vi "Get Index.vi"(7 "item":string, 8 "error in":errorcluster, 11 "[Items]":string[](array[string])) -> (0 "error out":errorcluster, 3 "index":i32)   [LabVIEW 2024, in "LV_OPC.lvlib"]
uses:
  LV_OPC.lvlib
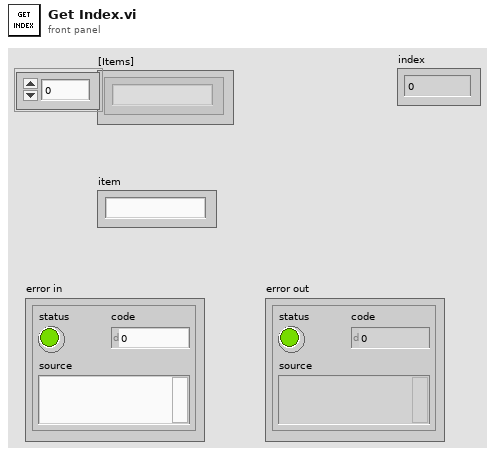
[diagram p1: front panel]
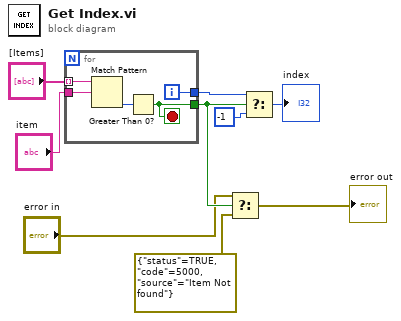
[diagram p0: block diagram]
diagram:
  n1 = for {
    tunnel: "[Items]" -> [w14] mode=indexing
    tunnel: [w12] -> w7
    tunnel: "item" -> [w11]
    tunnel: [w10] -> w4
    i -> [w12]
    stop <- w10 stop-if-true
    n2 = Match Pattern(string=w14, regular expression=w11) -> (offset past match=w13:i32)  [unwired: 1 in, 3 out]
    n3 = Greater Than 0?(x=w13) -> (x > 0?=w10:bool)
  }
  n4 = Select(t="error in", s=w4, f=errorcluster {"status"=TRUE, "code"=5000, "source"="Item Not found"}) -> (s? t:f=→"error out":errorcluster)
  n5 = Select(t=w7, s=w4, f=-1) -> (s? t:f=→"index":i32)
